vi "Write Dictionary.vi"(8 "error in (no error)":errorcluster, 10 "Dictionary":variant, 11 "CSSProperties in":refnum<class "CSSProperties.lvclass">) -> (0 "error out":errorcluster, 3 "CSSProperties out":refnum<class "CSSProperties.lvclass">)   [LabVIEW 2019, in "CSSProperties.lvclass"]
uses:
  CSSProperties.lvclass
  CSSProperties.lvclass/CSSProperties.ctl
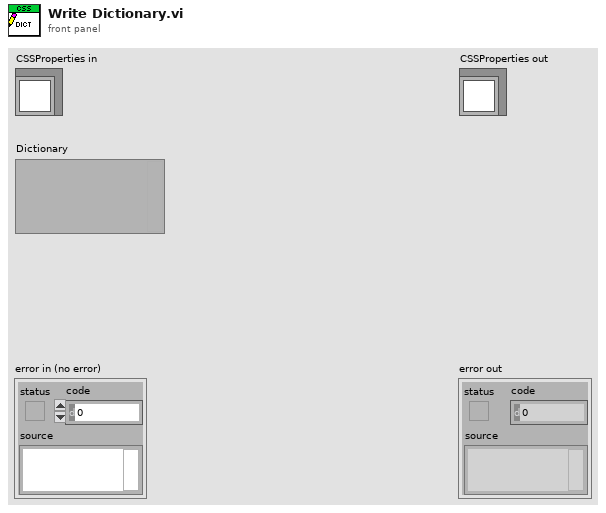
[diagram p1: front panel]
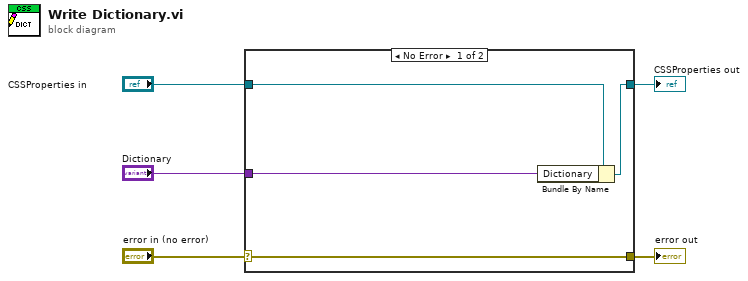
[diagram p0: block diagram]
diagram:
  n1 = case shown="No Error" "error in (no error)" {
    selector: "error in (no error)" -> [w9 w10]
    tunnel: [w9 w10] -> w4
    tunnel: [w7 w11] -> w2
    tunnel: "CSSProperties in" -> [w8 w11]
    tunnel: "Dictionary" -> [w6 _]
    frame No Error {
      n2 = Bundle By Name(cluster=w8, "Dictionary"=w6) -> (w7:refnum<class "CSSProperties.lvclass">)
    }
    frame Error {
    }
  }
  "error out" <- w4
  "CSSProperties out" <- w2
